vi "Test Error in RA DEC Conversions.vi"() -> ()   [LabVIEW 2021]
uses:
  typedefs/CC cluster RA and DEC.ctl
  Telescope/PRIME Telescope/PRIME Telescope.lvclass
panel:
  out "Array 2":dbl[](array[numeric])
  out "Array":dbl[](array[numeric])
  out "Waveform Graph 2":dbl[][](graph)
  out "Waveform Graph":dbl[][](graph)
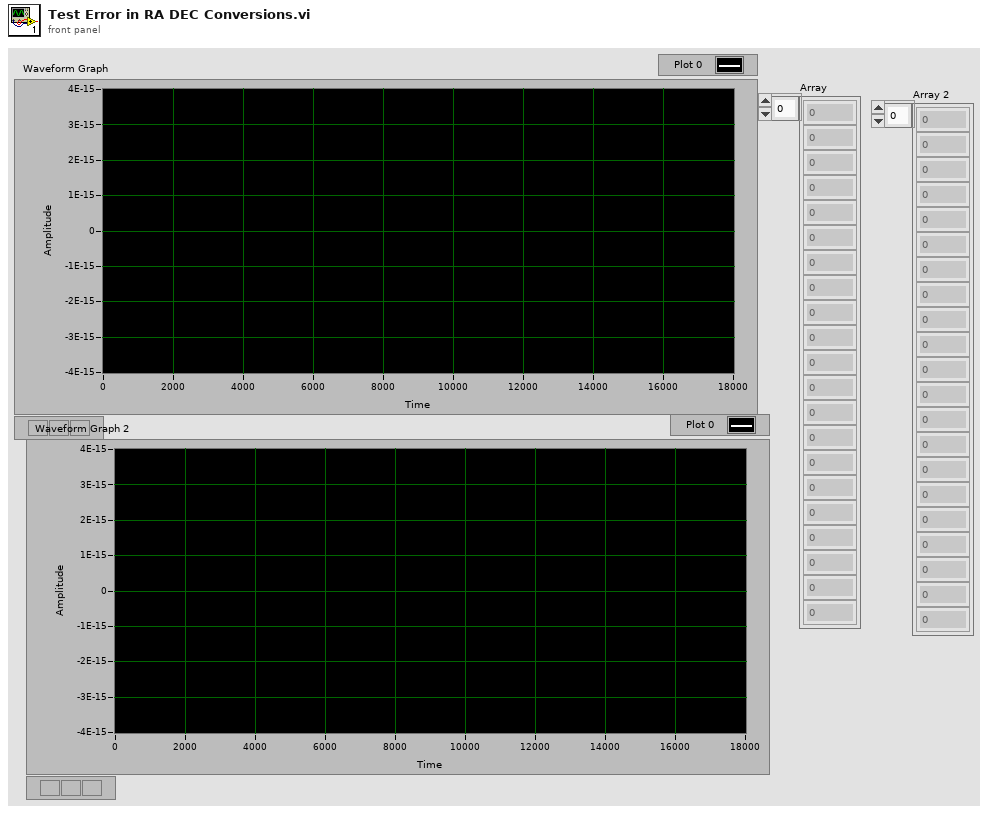
[diagram p1: front panel]
types:
  T1 = typedef "CC cluster RA and DEC.ctl" = cluster{"RA":dbl, "DEC":dbl}
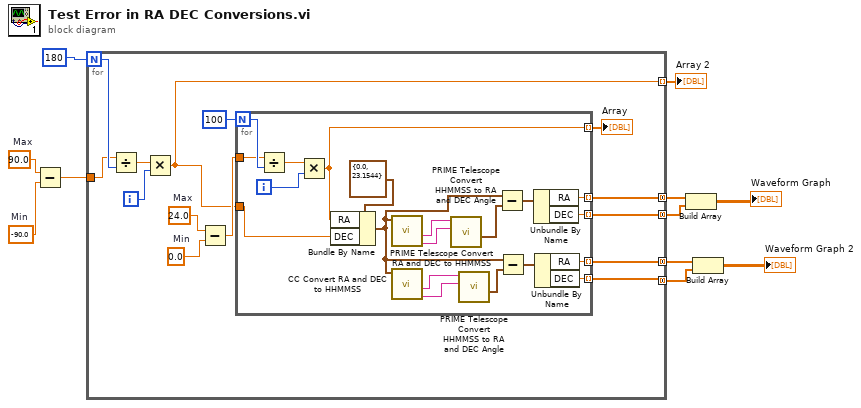
[diagram p0: block diagram]
diagram:
  w9 = 90.0  # Max
  w10 = -90.0  # Min
  n1 = Subtract(x=w9, y=w10) -> (x-y=w8:dbl)
  n2 = for {
    N: 180 -> [w24]
    tunnel: w8 -> [w23]
    tunnel: [w17] -> w7 mode=concatenating
    tunnel: [w16] -> w6 mode=concatenating
    tunnel: [w15] -> w4 mode=concatenating
    tunnel: [w14] -> w3 mode=concatenating
    tunnel: [w13] -> w1 mode=indexing
    i -> [w21]
    w19 = 24.0  # Max
    w20 = 0.0  # Min
    n3 = Divide(x=w23, y=w24) -> (x/y=w22:dbl)
    n4 = Multiply(x=w22, y=w21) -> (x*y=w13:dbl)
    n5 = Subtract(x=w19, y=w20) -> (x-y=w18:dbl)
    n6 = for {
      N: 100 -> [w45]
      tunnel: w18 -> [w44]
      tunnel: w13 -> [w40]
      tunnel: [w35] -> w17 mode=indexing
      tunnel: [w34] -> w16 mode=indexing
      tunnel: [w28] -> w15 mode=indexing
      tunnel: [w27] -> w14 mode=indexing
      tunnel: [w26] -> w12 mode=indexing
      i -> [w42]
      n7 = Divide(x=w44, y=w45) -> (x/y=w43:dbl)
      n8 = Multiply(x=w43, y=w42) -> (x*y=w26:dbl)
      n9 = Bundle By Name(cluster=T1 {"RA"=0.0, "DEC"=23.1544} ("RA and DEC"), "RA"=w26, "DEC"=w40) -> (w29:T1)
      n10 = call "PRIME Telescope Convert RA and DEC to HHMMSS.vi"("RA and DEC"=w29) -> ("Dec String"=w38:string, "RA String"=w39:string)  [unwired: 7 in, 2 out]
      n11 = call "CC Convert RA and DEC to HHMMSS.vi"("RA and DEC"=w29) -> ("DEC String"=w32:string, "RA String"=w33:string)  [unwired: 7 in, 2 out]
      n12 = call "PRIME Telescope Convert HHMMSS to RA and DEC Angle.vi"("Dec String"=w38, "RA String"=w39) -> ("RA and DEC"=w37:T1)  [unwired: 7 in, 2 out]
      n13 = call "PRIME Telescope Convert HHMMSS to RA and DEC Angle.vi"("Dec String"=w32, "RA String"=w33) -> ("RA and DEC"=w30:T1)  [unwired: 7 in, 2 out]
      n14 = Subtract(x=w29, y=w37) -> (x-y=w36:T1)
      n15 = Subtract(x=w29, y=w30) -> (x-y=w31:T1)
      n16 = Unbundle By Name(w36) -> ("RA"=w35:dbl, "DEC"=w34:dbl)
      n17 = Unbundle By Name(w31) -> ("RA"=w28:dbl, "DEC"=w27:dbl)
    }
    "Array" <- w12
  }
  "Array 2" <- w1
  n18 = Build Array(w7, w6) -> (→"Waveform Graph":dbl[][])
  n19 = Build Array(w4, w3) -> (→"Waveform Graph 2":dbl[][])
